vi "actividad_4.vi"() -> ()   [LabVIEW 2020]
panel:
  in  "stop":bool
  in  "Slide":dbl(slide) scale=0.0..50.0
  in  "Phase":dbl
  in  "Amplitude":dbl=1.0
  in  "Frequency":dbl=10.1
  in  "Reset Signal":bool
  out "Waveform Graph":dynamicdata(graph)
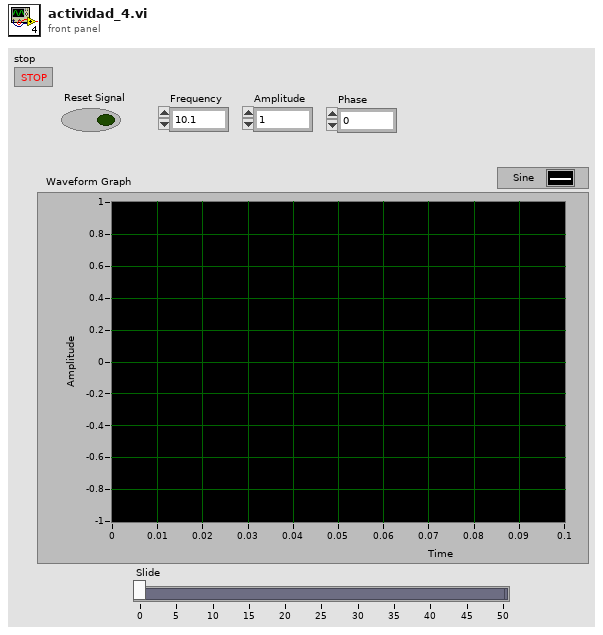
[diagram p1: front panel]
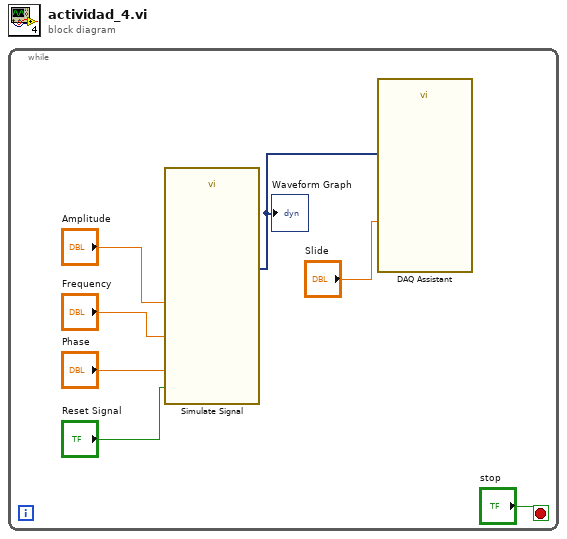
[diagram p0: block diagram]
diagram:
  n1 = while {
    stop <- "stop" stop-if-true
    n2 = call "Simulate Signal"("Reset Signal"="Reset Signal", "Frequency"="Frequency", "Amplitude"="Amplitude", "Phase"="Phase") -> ("Sine"=w7:dynamicdata)  [unwired: 10 in, 1 out]
    "Waveform Graph" <- w7
    n3 = call "DAQ Assistant"("data"=w7, "timeout (s)"="Slide") -> ()  [unwired: 16 in, 2 out]
  }
